vi "main(Test DQMH modules).vi"() -> ()   [LabVIEW 2018, in "Application.lvlib"] (continued)
                n5658 = To Variant(anything=T4."demux1_10_channel5" ("demux1_10(x6)_encode")) -> (Variant=w12358:variant)
                n5659 = To Variant(anything=bool[] [TRUE, FALSE, FALSE, FALSE, FALSE, FALSE]) -> (Variant=w12354:variant)
                n5660 = Bundle By Name(cluster=w12357, "command"="MEAS.AllRelaysOFF") -> (w12353:T9)
                n5661 = Bundle By Name(cluster=w12357, "command"="MEAS.mux10-1", "data"=w12364) -> (w12352:T9)
                n5662 = Bundle By Name(cluster=w12357, "command"="MEAS.mux6_1", "data"=w12362) -> (w12351:T9)
                n5663 = Bundle By Name(cluster=w12357, "command"="MEAS.demux1-10", "data"=w12358) -> (w12350:T9)
                n5664 = Bundle By Name(cluster=w12357, "command"="MEAS.eMIC", "data"=w12354) -> (w12349:T9)
                n5665 = Build Array(w12353, w12352, w12351, w12350, w12349) -> (w12334:T9[])
                n5666 = To Variant(anything=w12339) -> (Variant=w12337:variant)
                n5667 = To Variant(anything=w12339) -> (Variant=w12336:variant)
                n5668 = Bundle By Name(cluster=w12335, "command"="WaitFor") -> (w12333:T9)
                n5669 = Bundle By Name(cluster=w12335, "command"="MEAS.DMM dual read") -> (w12346:T9)
                n5670 = Bundle By Name(cluster=w12335, "command"="MEAS.requestAC", "data"=w12337) -> (w12345:T9)
                n5671 = Bundle By Name(cluster=w12335, "command"="Apps.WaitForEvent", "data"=w12336) -> (w12340:T9)
                n5672 = Bundle By Name(cluster=w12335, "command"="Apps.UI Update 1") -> (w12341:T9)
                n5673 = Build Array (concatenate)(w12334, w12333, w12346, w12345, w12340, w12341) -> (w12338:T9[])
              }
            }
          }
          frame True {
            n5674 = Bundle By Name(cluster=T9 {"command"="", "data"=variant} ("element"), "command"="Apps.UI Update 1") -> (w12368:T9)
            n5675 = Build Array(w12368) -> (w12367:T9[])
          }
        }
        n5676 = for {
          tunnel: w12283 -> [w12378] mode=indexing
          tunnel: w12291 -> [w12379]
          tunnel: [w12375] -> w12293 mode=indexing
          n5677 = Unbundle By Name(w12378) -> ("command"=w12377:string, "data"=w12376:variant)
          n5678 = call "App enquece.vi"("command data"=w12376, "command"=w12377, "queue in"=w12379) -> ("error out"=w12375:errorcluster)  [unwired: 7 in, 1 out]
        }
        n5679 = Merge Errors(w12294, w12293) -> (w12292:errorcluster)
      }
      frame "Test DRV 26A" {
        w12383 = 26 ("DUT index(0-59)")
        n5680 = disable-structure shown="LOGGING==TRUE" {
          disable-tunnel: w12388 -> [w12471 _]
          frame condition #0 (active) {
            n5681 = Empty String/Path?(string/path=w12471) -> (empty?=w12473:bool)
            n5682 = Select(t="Quece timeout", s=w12473, f=w12471) -> (s? t:f=w12470:string)
            n5683 = call "string log (SubVI).vi"("state Name"=w12470) -> ()  [unwired: 9 in, 2 out]
          }
          frame condition #1 {
          }
        }
        n5684 = Flush Queue(queue=w12389) -> (queue out=w12390:refnum<queue>)  [unwired: 1 in, 2 out]
        n5685 = Decrement(x=w12383) -> (x-1=w12387:i32)
        n5686 = Index Array(array=w12384, index=w12387) -> (element=w12385:refnum<vi>)
        n5687 = call "FGV DRV stand.vi"() -> ("Sub-Test.DCV"=w12380:bool)  [unwired: 10 in, 1 out]
        n5688 = call "FGV Driver Data.vi"("DUT index(1-60)"=w12383) -> ("DUT SC"=w12381:bool)  [unwired: 7 in, 3 out]
        n5689 = property class="ColBox"(reference=w12385, "Value"=u32 10000536 ("DRV 1")) -> ()  [unwired: 1 in, 2 out]
        n5690 = case shown="False" w12381 {
          tunnel: w12383 -> [w12401 _]
          tunnel: [w12400 w12466] -> w12382
          tunnel: w12380 -> [w12399 _]
          frame False {
            n5691 = case shown="False" w12399 {
              tunnel: w12401 -> [w12408 w12438]
              tunnel: [w12419 w12437] -> w12400
              frame False {
                w12405 = T9 {"command"="", "data"=variant} ("element")
                w12418 = T9 {"command"="", "data"=variant} ("element")
                n5692 = To Variant(anything=T3."mux10_1_channel5" ("mux10_1(x6)_encode")) -> (Variant=w12416:variant)
                n5693 = To Variant(anything=T4."demux1_10_channel5" ("demux1_10(x6)_encode")) -> (Variant=w12412:variant)
                n5694 = To Variant(anything=bool[] [FALSE, TRUE, FALSE, FALSE, FALSE, FALSE]) -> (Variant=w12427:variant)
                n5695 = Bundle By Name(cluster=w12418, "command"="MEAS.AllRelaysOFF") -> (w12426:T9)
                n5696 = Bundle By Name(cluster=w12418, "command"="MEAS.mux10-1", "data"=w12416) -> (w12409:T9)
                n5697 = Bundle By Name(cluster=w12418, "command"="MEAS.demux1-10", "data"=w12412) -> (w12410:T9)
                n5698 = Bundle By Name(cluster=w12418, "command"="MEAS.eMIC", "data"=w12427) -> (w12411:T9)
                n5699 = Build Array(w12426, w12409, w12410, w12411) -> (w12404:T9[])
                n5700 = To Variant(anything=w12408) -> (Variant=w12407:variant)
                n5701 = To Variant(anything=w12408) -> (Variant=w12406:variant)
                n5702 = Bundle By Name(cluster=w12405, "command"="MEAS.requestAC", "data"=w12407) -> (w12424:T9)
                n5703 = Bundle By Name(cluster=w12405, "command"="Apps.WaitForEvent", "data"=w12406) -> (w12420:T9)
                n5704 = Bundle By Name(cluster=w12405, "command"="Apps.UI Update 1") -> (w12421:T9)
                n5705 = Bundle By Name(cluster=w12405, "command"="WaitFor") -> (w12403:T9)
                n5706 = Build Array (concatenate)(w12404, w12403, w12424, w12420, w12421) -> (w12419:T9[])
              }
              frame True {
                w12434 = T9 {"command"="", "data"=variant} ("element")
                w12456 = T9 {"command"="", "data"=variant} ("element")
                n5707 = To Variant(anything=T3."mux10_1_channel5" ("mux10_1(x6)_encode")) -> (Variant=w12463:variant)
                n5708 = To Variant(anything=T2."mux6_1_channel2_3" ("mux6_1(3wires)_encode")) -> (Variant=w12461:variant)
                n5709 = To Variant(anything=T4."demux1_10_channel5" ("demux1_10(x6)_encode")) -> (Variant=w12457:variant)
                n5710 = To Variant(anything=bool[] [FALSE, TRUE, FALSE, FALSE, FALSE, FALSE]) -> (Variant=w12453:variant)
                n5711 = Bundle By Name(cluster=w12456, "command"="MEAS.AllRelaysOFF") -> (w12452:T9)
                n5712 = Bundle By Name(cluster=w12456, "command"="MEAS.mux10-1", "data"=w12463) -> (w12451:T9)
                n5713 = Bundle By Name(cluster=w12456, "command"="MEAS.mux6_1", "data"=w12461) -> (w12450:T9)
                n5714 = Bundle By Name(cluster=w12456, "command"="MEAS.demux1-10", "data"=w12457) -> (w12449:T9)
                n5715 = Bundle By Name(cluster=w12456, "command"="MEAS.eMIC", "data"=w12453) -> (w12448:T9)
                n5716 = Build Array(w12452, w12451, w12450, w12449, w12448) -> (w12433:T9[])
                n5717 = To Variant(anything=w12438) -> (Variant=w12436:variant)
                n5718 = To Variant(anything=w12438) -> (Variant=w12435:variant)
                n5719 = Bundle By Name(cluster=w12434, "command"="WaitFor") -> (w12432:T9)
                n5720 = Bundle By Name(cluster=w12434, "command"="MEAS.DMM dual read") -> (w12445:T9)
                n5721 = Bundle By Name(cluster=w12434, "command"="MEAS.requestAC", "data"=w12436) -> (w12444:T9)
                n5722 = Bundle By Name(cluster=w12434, "command"="Apps.WaitForEvent", "data"=w12435) -> (w12439:T9)
                n5723 = Bundle By Name(cluster=w12434, "command"="Apps.UI Update 1") -> (w12440:T9)
                n5724 = Build Array (concatenate)(w12433, w12432, w12445, w12444, w12439, w12440) -> (w12437:T9[])
              }
            }
          }
          frame True {
            n5725 = Bundle By Name(cluster=T9 {"command"="", "data"=variant} ("element"), "command"="Apps.UI Update 1") -> (w12467:T9)
            n5726 = Build Array(w12467) -> (w12466:T9[])
          }
        }
        n5727 = for {
          tunnel: w12382 -> [w12477] mode=indexing
          tunnel: w12390 -> [w12478]
          tunnel: [w12474] -> w12392 mode=indexing
          n5728 = Unbundle By Name(w12477) -> ("command"=w12476:string, "data"=w12475:variant)
          n5729 = call "App enquece.vi"("command data"=w12475, "command"=w12476, "queue in"=w12478) -> ("error out"=w12474:errorcluster)  [unwired: 7 in, 1 out]
        }
        n5730 = Merge Errors(w12393, w12392) -> (w12391:errorcluster)
      }
      frame "Test DRV 27A" {
        w12482 = 27 ("DUT index(0-59)")
        n5731 = disable-structure shown="LOGGING==TRUE" {
          disable-tunnel: w12487 -> [w12570 _]
          frame condition #0 (active) {
            n5732 = Empty String/Path?(string/path=w12570) -> (empty?=w12572:bool)
            n5733 = Select(t="Quece timeout", s=w12572, f=w12570) -> (s? t:f=w12569:string)
            n5734 = call "string log (SubVI).vi"("state Name"=w12569) -> ()  [unwired: 9 in, 2 out]
          }
          frame condition #1 {
          }
        }
        n5735 = Flush Queue(queue=w12488) -> (queue out=w12489:refnum<queue>)  [unwired: 1 in, 2 out]
        n5736 = Decrement(x=w12482) -> (x-1=w12486:i32)
        n5737 = Index Array(array=w12483, index=w12486) -> (element=w12484:refnum<vi>)
        n5738 = call "FGV DRV stand.vi"() -> ("Sub-Test.DCV"=w12479:bool)  [unwired: 10 in, 1 out]
        n5739 = call "FGV Driver Data.vi"("DUT index(1-60)"=w12482) -> ("DUT SC"=w12480:bool)  [unwired: 7 in, 3 out]
        n5740 = property class="ColBox"(reference=w12484, "Value"=u32 10000536 ("DRV 1")) -> ()  [unwired: 1 in, 2 out]
        n5741 = case shown="False" w12480 {
          tunnel: w12482 -> [w12500 _]
          tunnel: [w12499 w12565] -> w12481
          tunnel: w12479 -> [w12498 _]
          frame False {
            n5742 = case shown="True" w12498 {
              tunnel: w12500 -> [w12507 w12537]
              tunnel: [w12518 w12536] -> w12499
              frame False {
                w12504 = T9 {"command"="", "data"=variant} ("element")
                w12517 = T9 {"command"="", "data"=variant} ("element")
                n5743 = To Variant(anything=T3."mux10_1_channel5" ("mux10_1(x6)_encode")) -> (Variant=w12515:variant)
                n5744 = To Variant(anything=T4."demux1_10_channel5" ("demux1_10(x6)_encode")) -> (Variant=w12511:variant)
                n5745 = To Variant(anything=bool[] [FALSE, FALSE, TRUE, FALSE, FALSE, FALSE]) -> (Variant=w12526:variant)
                n5746 = Bundle By Name(cluster=w12517, "command"="MEAS.AllRelaysOFF") -> (w12525:T9)
                n5747 = Bundle By Name(cluster=w12517, "command"="MEAS.mux10-1", "data"=w12515) -> (w12508:T9)
                n5748 = Bundle By Name(cluster=w12517, "command"="MEAS.demux1-10", "data"=w12511) -> (w12509:T9)
                n5749 = Bundle By Name(cluster=w12517, "command"="MEAS.eMIC", "data"=w12526) -> (w12510:T9)
                n5750 = Build Array(w12525, w12508, w12509, w12510) -> (w12503:T9[])
                n5751 = To Variant(anything=w12507) -> (Variant=w12506:variant)
                n5752 = To Variant(anything=w12507) -> (Variant=w12505:variant)
                n5753 = Bundle By Name(cluster=w12504, "command"="MEAS.requestAC", "data"=w12506) -> (w12523:T9)
                n5754 = Bundle By Name(cluster=w12504, "command"="Apps.WaitForEvent", "data"=w12505) -> (w12519:T9)
                n5755 = Bundle By Name(cluster=w12504, "command"="Apps.UI Update 1") -> (w12520:T9)
                n5756 = Bundle By Name(cluster=w12504, "command"="WaitFor") -> (w12502:T9)
                n5757 = Build Array (concatenate)(w12503, w12502, w12523, w12519, w12520) -> (w12518:T9[])
              }
              frame True {
                w12533 = T9 {"command"="", "data"=variant} ("element")
                w12555 = T9 {"command"="", "data"=variant} ("element")
                n5758 = To Variant(anything=T3."mux10_1_channel5" ("mux10_1(x6)_encode")) -> (Variant=w12562:variant)
                n5759 = To Variant(anything=T2."mux6_1_channel3_3" ("mux6_1(3wires)_encode")) -> (Variant=w12560:variant)
                n5760 = To Variant(anything=T4."demux1_10_channel5" ("demux1_10(x6)_encode")) -> (Variant=w12556:variant)
                n5761 = To Variant(anything=bool[] [FALSE, FALSE, TRUE, FALSE, FALSE, FALSE]) -> (Variant=w12552:variant)
                n5762 = Bundle By Name(cluster=w12555, "command"="MEAS.AllRelaysOFF") -> (w12551:T9)
                n5763 = Bundle By Name(cluster=w12555, "command"="MEAS.mux10-1", "data"=w12562) -> (w12550:T9)
                n5764 = Bundle By Name(cluster=w12555, "command"="MEAS.mux6_1", "data"=w12560) -> (w12549:T9)
                n5765 = Bundle By Name(cluster=w12555, "command"="MEAS.demux1-10", "data"=w12556) -> (w12548:T9)
                n5766 = Bundle By Name(cluster=w12555, "command"="MEAS.eMIC", "data"=w12552) -> (w12547:T9)
                n5767 = Build Array(w12551, w12550, w12549, w12548, w12547) -> (w12532:T9[])
                n5768 = To Variant(anything=w12537) -> (Variant=w12535:variant)
                n5769 = To Variant(anything=w12537) -> (Variant=w12534:variant)
                n5770 = Bundle By Name(cluster=w12533, "command"="WaitFor") -> (w12531:T9)
                n5771 = Bundle By Name(cluster=w12533, "command"="MEAS.DMM dual read") -> (w12544:T9)
                n5772 = Bundle By Name(cluster=w12533, "command"="MEAS.requestAC", "data"=w12535) -> (w12543:T9)
                n5773 = Bundle By Name(cluster=w12533, "command"="Apps.WaitForEvent", "data"=w12534) -> (w12538:T9)
                n5774 = Bundle By Name(cluster=w12533, "command"="Apps.UI Update 1") -> (w12539:T9)
                n5775 = Build Array (concatenate)(w12532, w12531, w12544, w12543, w12538, w12539) -> (w12536:T9[])
              }
            }
          }
          frame True {
            n5776 = Bundle By Name(cluster=T9 {"command"="", "data"=variant} ("element"), "command"="Apps.UI Update 1") -> (w12566:T9)
            n5777 = Build Array(w12566) -> (w12565:T9[])
          }
        }
        n5778 = for {
          tunnel: w12481 -> [w12576] mode=indexing
          tunnel: w12489 -> [w12577]
          tunnel: [w12573] -> w12491 mode=indexing
          n5779 = Unbundle By Name(w12576) -> ("command"=w12575:string, "data"=w12574:variant)
          n5780 = call "App enquece.vi"("command data"=w12574, "command"=w12575, "queue in"=w12577) -> ("error out"=w12573:errorcluster)  [unwired: 7 in, 1 out]
        }
        n5781 = Merge Errors(w12492, w12491) -> (w12490:errorcluster)
      }
      frame "Test DRV 28A" {
        w12581 = 28 ("DUT index(0-59)")
        n5782 = disable-structure shown="LOGGING==TRUE" {
          disable-tunnel: w12586 -> [w12669 _]
          frame condition #0 (active) {
            n5783 = Empty String/Path?(string/path=w12669) -> (empty?=w12671:bool)
            n5784 = Select(t="Quece timeout", s=w12671, f=w12669) -> (s? t:f=w12668:string)
            n5785 = call "string log (SubVI).vi"("state Name"=w12668) -> ()  [unwired: 9 in, 2 out]
          }
          frame condition #1 {
          }
        }
        n5786 = Flush Queue(queue=w12587) -> (queue out=w12588:refnum<queue>)  [unwired: 1 in, 2 out]
        n5787 = Decrement(x=w12581) -> (x-1=w12585:i32)
        n5788 = Index Array(array=w12582, index=w12585) -> (element=w12583:refnum<vi>)
        n5789 = call "FGV DRV stand.vi"() -> ("Sub-Test.DCV"=w12578:bool)  [unwired: 10 in, 1 out]
        n5790 = call "FGV Driver Data.vi"("DUT index(1-60)"=w12581) -> ("DUT SC"=w12579:bool)  [unwired: 7 in, 3 out]
        n5791 = property class="ColBox"(reference=w12583, "Value"=u32 10000536 ("DRV 1")) -> ()  [unwired: 1 in, 2 out]
        n5792 = case shown="False" w12579 {
          tunnel: w12581 -> [w12599 _]
          tunnel: [w12598 w12664] -> w12580
          tunnel: w12578 -> [w12597 _]
          frame False {
            n5793 = case shown="False" w12597 {
              tunnel: w12599 -> [w12606 w12636]
              tunnel: [w12617 w12635] -> w12598
              frame False {
                w12603 = T9 {"command"="", "data"=variant} ("element")
                w12616 = T9 {"command"="", "data"=variant} ("element")
                n5794 = To Variant(anything=T3."mux10_1_channel5" ("mux10_1(x6)_encode")) -> (Variant=w12614:variant)
                n5795 = To Variant(anything=T4."demux1_10_channel5" ("demux1_10(x6)_encode")) -> (Variant=w12610:variant)
                n5796 = To Variant(anything=bool[] [FALSE, FALSE, FALSE, TRUE, FALSE, FALSE]) -> (Variant=w12625:variant)
                n5797 = Bundle By Name(cluster=w12616, "command"="MEAS.AllRelaysOFF") -> (w12624:T9)
                n5798 = Bundle By Name(cluster=w12616, "command"="MEAS.mux10-1", "data"=w12614) -> (w12607:T9)
                n5799 = Bundle By Name(cluster=w12616, "command"="MEAS.demux1-10", "data"=w12610) -> (w12608:T9)
                n5800 = Bundle By Name(cluster=w12616, "command"="MEAS.eMIC", "data"=w12625) -> (w12609:T9)
                n5801 = Build Array(w12624, w12607, w12608, w12609) -> (w12602:T9[])
                n5802 = To Variant(anything=w12606) -> (Variant=w12605:variant)
                n5803 = To Variant(anything=w12606) -> (Variant=w12604:variant)
                n5804 = Bundle By Name(cluster=w12603, "command"="MEAS.requestAC", "data"=w12605) -> (w12622:T9)
                n5805 = Bundle By Name(cluster=w12603, "command"="Apps.WaitForEvent", "data"=w12604) -> (w12618:T9)
                n5806 = Bundle By Name(cluster=w12603, "command"="Apps.UI Update 1") -> (w12619:T9)
                n5807 = Bundle By Name(cluster=w12603, "command"="WaitFor") -> (w12601:T9)
                n5808 = Build Array (concatenate)(w12602, w12601, w12622, w12618, w12619) -> (w12617:T9[])
              }
              frame True {
                w12632 = T9 {"command"="", "data"=variant} ("element")
                w12654 = T9 {"command"="", "data"=variant} ("element")
                n5809 = To Variant(anything=T3."mux10_1_channel5" ("mux10_1(x6)_encode")) -> (Variant=w12661:variant)
                n5810 = To Variant(anything=T2."mux6_1_channel4_3" ("mux6_1(3wires)_encode")) -> (Variant=w12659:variant)
                n5811 = To Variant(anything=T4."demux1_10_channel5" ("demux1_10(x6)_encode")) -> (Variant=w12655:variant)
                n5812 = To Variant(anything=bool[] [FALSE, FALSE, FALSE, TRUE, FALSE, FALSE]) -> (Variant=w12651:variant)
                n5813 = Bundle By Name(cluster=w12654, "command"="MEAS.AllRelaysOFF") -> (w12650:T9)
                n5814 = Bundle By Name(cluster=w12654, "command"="MEAS.mux10-1", "data"=w12661) -> (w12649:T9)
                n5815 = Bundle By Name(cluster=w12654, "command"="MEAS.mux6_1", "data"=w12659) -> (w12648:T9)
                n5816 = Bundle By Name(cluster=w12654, "command"="MEAS.demux1-10", "data"=w12655) -> (w12647:T9)
                n5817 = Bundle By Name(cluster=w12654, "command"="MEAS.eMIC", "data"=w12651) -> (w12646:T9)
                n5818 = Build Array(w12650, w12649, w12648, w12647, w12646) -> (w12631:T9[])
                n5819 = To Variant(anything=w12636) -> (Variant=w12634:variant)
                n5820 = To Variant(anything=w12636) -> (Variant=w12633:variant)
                n5821 = Bundle By Name(cluster=w12632, "command"="WaitFor") -> (w12630:T9)
                n5822 = Bundle By Name(cluster=w12632, "command"="MEAS.DMM dual read") -> (w12643:T9)
                n5823 = Bundle By Name(cluster=w12632, "command"="MEAS.requestAC", "data"=w12634) -> (w12642:T9)
                n5824 = Bundle By Name(cluster=w12632, "command"="Apps.WaitForEvent", "data"=w12633) -> (w12637:T9)
                n5825 = Bundle By Name(cluster=w12632, "command"="Apps.UI Update 1") -> (w12638:T9)
                n5826 = Build Array (concatenate)(w12631, w12630, w12643, w12642, w12637, w12638) -> (w12635:T9[])
              }
            }
          }
          frame True {
            n5827 = Bundle By Name(cluster=T9 {"command"="", "data"=variant} ("element"), "command"="Apps.UI Update 1") -> (w12665:T9)
            n5828 = Build Array(w12665) -> (w12664:T9[])
          }
        }
        n5829 = for {
          tunnel: w12580 -> [w12675] mode=indexing
          tunnel: w12588 -> [w12676]
          tunnel: [w12672] -> w12590 mode=indexing
          n5830 = Unbundle By Name(w12675) -> ("command"=w12674:string, "data"=w12673:variant)
          n5831 = call "App enquece.vi"("command data"=w12673, "command"=w12674, "queue in"=w12676) -> ("error out"=w12672:errorcluster)  [unwired: 7 in, 1 out]
        }
        n5832 = Merge Errors(w12591, w12590) -> (w12589:errorcluster)
      }
      frame "Test DRV 29A" {
        w12680 = 29 ("DUT index(0-59)")
        n5833 = disable-structure shown="LOGGING==TRUE" {
          disable-tunnel: w12685 -> [w12768 _]
          frame condition #0 (active) {
            n5834 = Empty String/Path?(string/path=w12768) -> (empty?=w12770:bool)
            n5835 = Select(t="Quece timeout", s=w12770, f=w12768) -> (s? t:f=w12767:string)
            n5836 = call "string log (SubVI).vi"("state Name"=w12767) -> ()  [unwired: 9 in, 2 out]
          }
          frame condition #1 {
          }
        }
        n5837 = Flush Queue(queue=w12686) -> (queue out=w12687:refnum<queue>)  [unwired: 1 in, 2 out]
        n5838 = Decrement(x=w12680) -> (x-1=w12684:i32)
        n5839 = Index Array(array=w12681, index=w12684) -> (element=w12682:refnum<vi>)
        n5840 = call "FGV DRV stand.vi"() -> ("Sub-Test.DCV"=w12677:bool)  [unwired: 10 in, 1 out]
        n5841 = call "FGV Driver Data.vi"("DUT index(1-60)"=w12680) -> ("DUT SC"=w12678:bool)  [unwired: 7 in, 3 out]
        n5842 = property class="ColBox"(reference=w12682, "Value"=u32 10000536 ("DRV 1")) -> ()  [unwired: 1 in, 2 out]
        n5843 = case shown="False" w12678 {
          tunnel: w12680 -> [w12698 _]
          tunnel: [w12697 w12763] -> w12679
          tunnel: w12677 -> [w12696 _]
          frame False {
            n5844 = case shown="True" w12696 {
              tunnel: w12698 -> [w12705 w12735]
              tunnel: [w12716 w12734] -> w12697
              frame False {
                w12702 = T9 {"command"="", "data"=variant} ("element")
                w12715 = T9 {"command"="", "data"=variant} ("element")
                n5845 = To Variant(anything=T3."mux10_1_channel5" ("mux10_1(x6)_encode")) -> (Variant=w12713:variant)
                n5846 = To Variant(anything=T4."demux1_10_channel5" ("demux1_10(x6)_encode")) -> (Variant=w12709:variant)
                n5847 = To Variant(anything=bool[] [FALSE, FALSE, FALSE, FALSE, TRUE, FALSE]) -> (Variant=w12724:variant)
                n5848 = Bundle By Name(cluster=w12715, "command"="MEAS.AllRelaysOFF") -> (w12723:T9)
                n5849 = Bundle By Name(cluster=w12715, "command"="MEAS.mux10-1", "data"=w12713) -> (w12706:T9)
                n5850 = Bundle By Name(cluster=w12715, "command"="MEAS.demux1-10", "data"=w12709) -> (w12707:T9)
                n5851 = Bundle By Name(cluster=w12715, "command"="MEAS.eMIC", "data"=w12724) -> (w12708:T9)
                n5852 = Build Array(w12723, w12706, w12707, w12708) -> (w12701:T9[])
                n5853 = To Variant(anything=w12705) -> (Variant=w12704:variant)
                n5854 = To Variant(anything=w12705) -> (Variant=w12703:variant)
                n5855 = Bundle By Name(cluster=w12702, "command"="MEAS.requestAC", "data"=w12704) -> (w12721:T9)
                n5856 = Bundle By Name(cluster=w12702, "command"="Apps.WaitForEvent", "data"=w12703) -> (w12717:T9)
                n5857 = Bundle By Name(cluster=w12702, "command"="Apps.UI Update 1") -> (w12718:T9)
                n5858 = Bundle By Name(cluster=w12702, "command"="WaitFor") -> (w12700:T9)
                n5859 = Build Array (concatenate)(w12701, w12700, w12721, w12717, w12718) -> (w12716:T9[])
              }
              frame True {
                w12731 = T9 {"command"="", "data"=variant} ("element")
                w12753 = T9 {"command"="", "data"=variant} ("element")
                n5860 = To Variant(anything=T3."mux10_1_channel5" ("mux10_1(x6)_encode")) -> (Variant=w12760:variant)
                n5861 = To Variant(anything=T2."mux6_1_channel5_3" ("mux6_1(3wires)_encode")) -> (Variant=w12758:variant)
                n5862 = To Variant(anything=T4."demux1_10_channel5" ("demux1_10(x6)_encode")) -> (Variant=w12754:variant)
                n5863 = To Variant(anything=bool[] [FALSE, FALSE, FALSE, FALSE, TRUE, FALSE]) -> (Variant=w12750:variant)
                n5864 = Bundle By Name(cluster=w12753, "command"="MEAS.AllRelaysOFF") -> (w12749:T9)
                n5865 = Bundle By Name(cluster=w12753, "command"="MEAS.mux10-1", "data"=w12760) -> (w12748:T9)
                n5866 = Bundle By Name(cluster=w12753, "command"="MEAS.mux6_1", "data"=w12758) -> (w12747:T9)
                n5867 = Bundle By Name(cluster=w12753, "command"="MEAS.demux1-10", "data"=w12754) -> (w12746:T9)
                n5868 = Bundle By Name(cluster=w12753, "command"="MEAS.eMIC", "data"=w12750) -> (w12745:T9)
                n5869 = Build Array(w12749, w12748, w12747, w12746, w12745) -> (w12730:T9[])
                n5870 = To Variant(anything=w12735) -> (Variant=w12733:variant)
                n5871 = To Variant(anything=w12735) -> (Variant=w12732:variant)
                n5872 = Bundle By Name(cluster=w12731, "command"="WaitFor") -> (w12729:T9)
                n5873 = Bundle By Name(cluster=w12731, "command"="MEAS.DMM dual read") -> (w12742:T9)
                n5874 = Bundle By Name(cluster=w12731, "command"="MEAS.requestAC", "data"=w12733) -> (w12741:T9)
                n5875 = Bundle By Name(cluster=w12731, "command"="Apps.WaitForEvent", "data"=w12732) -> (w12736:T9)
                n5876 = Bundle By Name(cluster=w12731, "command"="Apps.UI Update 1") -> (w12737:T9)
                n5877 = Build Array (concatenate)(w12730, w12729, w12742, w12741, w12736, w12737) -> (w12734:T9[])
              }
            }
          }
          frame True {
            n5878 = Bundle By Name(cluster=T9 {"command"="", "data"=variant} ("element"), "command"="Apps.UI Update 1") -> (w12764:T9)
            n5879 = Build Array(w12764) -> (w12763:T9[])
          }
        }
        n5880 = for {
          tunnel: w12679 -> [w12774] mode=indexing
          tunnel: w12687 -> [w12775]
          tunnel: [w12771] -> w12689 mode=indexing
          n5881 = Unbundle By Name(w12774) -> ("command"=w12773:string, "data"=w12772:variant)
          n5882 = call "App enquece.vi"("command data"=w12772, "command"=w12773, "queue in"=w12775) -> ("error out"=w12771:errorcluster)  [unwired: 7 in, 1 out]
        }
        n5883 = Merge Errors(w12690, w12689) -> (w12688:errorcluster)
      }
      frame "Test DRV 30A" {
        w12779 = 30 ("DUT index(0-59)")
        n5884 = disable-structure shown="LOGGING==TRUE" {
          disable-tunnel: w12784 -> [w12867 _]
          frame condition #0 (active) {
            n5885 = Empty String/Path?(string/path=w12867) -> (empty?=w12869:bool)
            n5886 = Select(t="Quece timeout", s=w12869, f=w12867) -> (s? t:f=w12866:string)
            n5887 = call "string log (SubVI).vi"("state Name"=w12866) -> ()  [unwired: 9 in, 2 out]
          }
          frame condition #1 {
          }
        }
        n5888 = Flush Queue(queue=w12785) -> (queue out=w12786:refnum<queue>)  [unwired: 1 in, 2 out]
        n5889 = Decrement(x=w12779) -> (x-1=w12783:i32)
        n5890 = Index Array(array=w12780, index=w12783) -> (element=w12781:refnum<vi>)
        n5891 = call "FGV DRV stand.vi"() -> ("Sub-Test.DCV"=w12776:bool)  [unwired: 10 in, 1 out]
        n5892 = call "FGV Driver Data.vi"("DUT index(1-60)"=w12779) -> ("DUT SC"=w12777:bool)  [unwired: 7 in, 3 out]
        n5893 = property class="ColBox"(reference=w12781, "Value"=u32 10000536 ("DRV 1")) -> ()  [unwired: 1 in, 2 out]
        n5894 = case shown="False" w12777 {
          tunnel: w12779 -> [w12797 _]
          tunnel: [w12796 w12862] -> w12778
          tunnel: w12776 -> [w12795 _]
          frame False {
            n5895 = case shown="False" w12795 {
              tunnel: w12797 -> [w12804 w12834]
              tunnel: [w12815 w12833] -> w12796
              frame False {
                w12801 = T9 {"command"="", "data"=variant} ("element")
                w12814 = T9 {"command"="", "data"=variant} ("element")
                n5896 = To Variant(anything=T3."mux10_1_channel5" ("mux10_1(x6)_encode")) -> (Variant=w12812:variant)
                n5897 = To Variant(anything=T4."demux1_10_channel5" ("demux1_10(x6)_encode")) -> (Variant=w12808:variant)
                n5898 = To Variant(anything=bool[] [FALSE, FALSE, FALSE, FALSE, FALSE, TRUE]) -> (Variant=w12823:variant)
                n5899 = Bundle By Name(cluster=w12814, "command"="MEAS.AllRelaysOFF") -> (w12822:T9)
                n5900 = Bundle By Name(cluster=w12814, "command"="MEAS.mux10-1", "data"=w12812) -> (w12805:T9)
                n5901 = Bundle By Name(cluster=w12814, "command"="MEAS.demux1-10", "data"=w12808) -> (w12806:T9)
                n5902 = Bundle By Name(cluster=w12814, "command"="MEAS.eMIC", "data"=w12823) -> (w12807:T9)
                n5903 = Build Array(w12822, w12805, w12806, w12807) -> (w12800:T9[])
                n5904 = To Variant(anything=w12804) -> (Variant=w12803:variant)
                n5905 = To Variant(anything=w12804) -> (Variant=w12802:variant)
                n5906 = Bundle By Name(cluster=w12801, "command"="MEAS.requestAC", "data"=w12803) -> (w12820:T9)
                n5907 = Bundle By Name(cluster=w12801, "command"="Apps.WaitForEvent", "data"=w12802) -> (w12816:T9)
                n5908 = Bundle By Name(cluster=w12801, "command"="Apps.UI Update 1") -> (w12817:T9)
                n5909 = Bundle By Name(cluster=w12801, "command"="WaitFor") -> (w12799:T9)
                n5910 = Build Array (concatenate)(w12800, w12799, w12820, w12816, w12817) -> (w12815:T9[])
              }
              frame True {
                w12830 = T9 {"command"="", "data"=variant} ("element")
                w12852 = T9 {"command"="", "data"=variant} ("element")
                n5911 = To Variant(anything=T3."mux10_1_channel5" ("mux10_1(x6)_encode")) -> (Variant=w12859:variant)
                n5912 = To Variant(anything=T2."mux6_1_channel6_3" ("mux6_1(3wires)_encode")) -> (Variant=w12857:variant)
                n5913 = To Variant(anything=T4."demux1_10_channel5" ("demux1_10(x6)_encode")) -> (Variant=w12853:variant)
                n5914 = To Variant(anything=bool[] [FALSE, FALSE, FALSE, FALSE, FALSE, TRUE]) -> (Variant=w12849:variant)
                n5915 = Bundle By Name(cluster=w12852, "command"="MEAS.AllRelaysOFF") -> (w12848:T9)
                n5916 = Bundle By Name(cluster=w12852, "command"="MEAS.mux10-1", "data"=w12859) -> (w12847:T9)
                n5917 = Bundle By Name(cluster=w12852, "command"="MEAS.mux6_1", "data"=w12857) -> (w12846:T9)
                n5918 = Bundle By Name(cluster=w12852, "command"="MEAS.demux1-10", "data"=w12853) -> (w12845:T9)
                n5919 = Bundle By Name(cluster=w12852, "command"="MEAS.eMIC", "data"=w12849) -> (w12844:T9)
                n5920 = Build Array(w12848, w12847, w12846, w12845, w12844) -> (w12829:T9[])
                n5921 = To Variant(anything=w12834) -> (Variant=w12832:variant)
                n5922 = To Variant(anything=w12834) -> (Variant=w12831:variant)
                n5923 = Bundle By Name(cluster=w12830, "command"="WaitFor") -> (w12828:T9)
                n5924 = Bundle By Name(cluster=w12830, "command"="MEAS.DMM dual read") -> (w12841:T9)
                n5925 = Bundle By Name(cluster=w12830, "command"="MEAS.requestAC", "data"=w12832) -> (w12840:T9)
                n5926 = Bundle By Name(cluster=w12830, "command"="Apps.WaitForEvent", "data"=w12831) -> (w12835:T9)
                n5927 = Bundle By Name(cluster=w12830, "command"="Apps.UI Update 1") -> (w12836:T9)
                n5928 = Build Array (concatenate)(w12829, w12828, w12841, w12840, w12835, w12836) -> (w12833:T9[])
              }
            }
          }
          frame True {
            n5929 = Bundle By Name(cluster=T9 {"command"="", "data"=variant} ("element"), "command"="Apps.UI Update 1") -> (w12863:T9)
            n5930 = Build Array(w12863) -> (w12862:T9[])
          }
        }
        n5931 = for {
          tunnel: w12778 -> [w12873] mode=indexing
          tunnel: w12786 -> [w12874]
          tunnel: [w12870] -> w12788 mode=indexing
          n5932 = Unbundle By Name(w12873) -> ("command"=w12872:string, "data"=w12871:variant)
          n5933 = call "App enquece.vi"("command data"=w12871, "command"=w12872, "queue in"=w12874) -> ("error out"=w12870:errorcluster)  [unwired: 7 in, 1 out]
        }
        n5934 = Merge Errors(w12789, w12788) -> (w12787:errorcluster)
      }
      frame "Test DRV 31A" {
        w12878 = 31 ("DUT index(0-59)")
        n5935 = disable-structure shown="LOGGING==TRUE" {
          disable-tunnel: w12883 -> [w12966 _]
          frame condition #0 (active) {
            n5936 = Empty String/Path?(string/path=w12966) -> (empty?=w12968:bool)
            n5937 = Select(t="Quece timeout", s=w12968, f=w12966) -> (s? t:f=w12965:string)
            n5938 = call "string log (SubVI).vi"("state Name"=w12965) -> ()  [unwired: 9 in, 2 out]
          }
          frame condition #1 {
          }
        }
        n5939 = Flush Queue(queue=w12884) -> (queue out=w12885:refnum<queue>)  [unwired: 1 in, 2 out]
        n5940 = Decrement(x=w12878) -> (x-1=w12882:i32)
        n5941 = Index Array(array=w12879, index=w12882) -> (element=w12880:refnum<vi>)
        n5942 = call "FGV DRV stand.vi"() -> ("Sub-Test.DCV"=w12875:bool)  [unwired: 10 in, 1 out]
        n5943 = call "FGV Driver Data.vi"("DUT index(1-60)"=w12878) -> ("DUT SC"=w12876:bool)  [unwired: 7 in, 3 out]
        n5944 = property class="ColBox"(reference=w12880, "Value"=u32 10000536 ("DRV 1")) -> ()  [unwired: 1 in, 2 out]
        n5945 = case shown="False" w12876 {
          tunnel: w12878 -> [w12896 _]
          tunnel: [w12895 w12961] -> w12877
          tunnel: w12875 -> [w12894 _]
          frame False {
            n5946 = case shown="True" w12894 {
              tunnel: w12896 -> [w12903 w12933]
              tunnel: [w12914 w12932] -> w12895
              frame False {
                w12900 = T9 {"command"="", "data"=variant} ("element")
                w12913 = T9 {"command"="", "data"=variant} ("element")
                n5947 = To Variant(anything=T3."mux10_1_channel6" ("mux10_1(x6)_encode")) -> (Variant=w12911:variant)
                n5948 = To Variant(anything=T4."demux1_10_channel6" ("demux1_10(x6)_encode")) -> (Variant=w12907:variant)
                n5949 = To Variant(anything=bool[] [TRUE, FALSE, FALSE, FALSE, FALSE, FALSE]) -> (Variant=w12922:variant)
                n5950 = Bundle By Name(cluster=w12913, "command"="MEAS.AllRelaysOFF") -> (w12921:T9)
                n5951 = Bundle By Name(cluster=w12913, "command"="MEAS.mux10-1", "data"=w12911) -> (w12904:T9)
                n5952 = Bundle By Name(cluster=w12913, "command"="MEAS.demux1-10", "data"=w12907) -> (w12905:T9)
                n5953 = Bundle By Name(cluster=w12913, "command"="MEAS.eMIC", "data"=w12922) -> (w12906:T9)
                n5954 = Build Array(w12921, w12904, w12905, w12906) -> (w12899:T9[])
                n5955 = To Variant(anything=w12903) -> (Variant=w12902:variant)
                n5956 = To Variant(anything=w12903) -> (Variant=w12901:variant)
                n5957 = Bundle By Name(cluster=w12900, "command"="MEAS.requestAC", "data"=w12902) -> (w12919:T9)
                n5958 = Bundle By Name(cluster=w12900, "command"="Apps.WaitForEvent", "data"=w12901) -> (w12915:T9)
                n5959 = Bundle By Name(cluster=w12900, "command"="Apps.UI Update 1") -> (w12916:T9)
                n5960 = Bundle By Name(cluster=w12900, "command"="WaitFor") -> (w12898:T9)
                n5961 = Build Array (concatenate)(w12899, w12898, w12919, w12915, w12916) -> (w12914:T9[])
              }
              frame True {
                w12929 = T9 {"command"="", "data"=variant} ("element")
                w12951 = T9 {"command"="", "data"=variant} ("element")
                n5962 = To Variant(anything=T3."mux10_1_channel6" ("mux10_1(x6)_encode")) -> (Variant=w12958:variant)
                n5963 = To Variant(anything=T2."mux6_1_channel1_3" ("mux6_1(3wires)_encode")) -> (Variant=w12956:variant)
                n5964 = To Variant(anything=T4."demux1_10_channel6" ("demux1_10(x6)_encode")) -> (Variant=w12952:variant)
                n5965 = To Variant(anything=bool[] [TRUE, FALSE, FALSE, FALSE, FALSE, FALSE]) -> (Variant=w12948:variant)
                n5966 = Bundle By Name(cluster=w12951, "command"="MEAS.AllRelaysOFF") -> (w12947:T9)
                n5967 = Bundle By Name(cluster=w12951, "command"="MEAS.mux10-1", "data"=w12958) -> (w12946:T9)
                n5968 = Bundle By Name(cluster=w12951, "command"="MEAS.mux6_1", "data"=w12956) -> (w12945:T9)
                n5969 = Bundle By Name(cluster=w12951, "command"="MEAS.demux1-10", "data"=w12952) -> (w12944:T9)
                n5970 = Bundle By Name(cluster=w12951, "command"="MEAS.eMIC", "data"=w12948) -> (w12943:T9)
                n5971 = Build Array(w12947, w12946, w12945, w12944, w12943) -> (w12928:T9[])
                n5972 = To Variant(anything=w12933) -> (Variant=w12931:variant)
                n5973 = To Variant(anything=w12933) -> (Variant=w12930:variant)
                n5974 = Bundle By Name(cluster=w12929, "command"="WaitFor") -> (w12927:T9)
                n5975 = Bundle By Name(cluster=w12929, "command"="MEAS.DMM dual read") -> (w12940:T9)
                n5976 = Bundle By Name(cluster=w12929, "command"="MEAS.requestAC", "data"=w12931) -> (w12939:T9)
                n5977 = Bundle By Name(cluster=w12929, "command"="Apps.WaitForEvent", "data"=w12930) -> (w12934:T9)
                n5978 = Bundle By Name(cluster=w12929, "command"="Apps.UI Update 1") -> (w12935:T9)
                n5979 = Build Array (concatenate)(w12928, w12927, w12940, w12939, w12934, w12935) -> (w12932:T9[])
              }
            }
          }
          frame True {
            n5980 = Bundle By Name(cluster=T9 {"command"="", "data"=variant} ("element"), "command"="Apps.UI Update 1") -> (w12962:T9)
            n5981 = Build Array(w12962) -> (w12961:T9[])
          }
        }
        n5982 = for {
          tunnel: w12877 -> [w12972] mode=indexing
          tunnel: w12885 -> [w12973]
          tunnel: [w12969] -> w12887 mode=indexing
          n5983 = Unbundle By Name(w12972) -> ("command"=w12971:string, "data"=w12970:variant)
          n5984 = call "App enquece.vi"("command data"=w12970, "command"=w12971, "queue in"=w12973) -> ("error out"=w12969:errorcluster)  [unwired: 7 in, 1 out]
        }
        n5985 = Merge Errors(w12888, w12887) -> (w12886:errorcluster)
      }
      frame "Test DRV 32A" {
        w12977 = 32 ("DUT index(0-59)")
        n5986 = disable-structure shown="LOGGING==TRUE" {
          disable-tunnel: w12982 -> [w13065 _]
          frame condition #0 (active) {
            n5987 = Empty String/Path?(string/path=w13065) -> (empty?=w13067:bool)
            n5988 = Select(t="Quece timeout", s=w13067, f=w13065) -> (s? t:f=w13064:string)
            n5989 = call "string log (SubVI).vi"("state Name"=w13064) -> ()  [unwired: 9 in, 2 out]
          }
          frame condition #1 {
          }
        }
        n5990 = Flush Queue(queue=w12983) -> (queue out=w12984:refnum<queue>)  [unwired: 1 in, 2 out]
        n5991 = Decrement(x=w12977) -> (x-1=w12981:i32)
        n5992 = Index Array(array=w12978, index=w12981) -> (element=w12979:refnum<vi>)
        n5993 = call "FGV DRV stand.vi"() -> ("Sub-Test.DCV"=w12974:bool)  [unwired: 10 in, 1 out]
        n5994 = call "FGV Driver Data.vi"("DUT index(1-60)"=w12977) -> ("DUT SC"=w12975:bool)  [unwired: 7 in, 3 out]
        n5995 = property class="ColBox"(reference=w12979, "Value"=u32 10000536 ("DRV 1")) -> ()  [unwired: 1 in, 2 out]
        n5996 = case shown="False" w12975 {
          tunnel: w12977 -> [w12995 _]
          tunnel: [w12994 w13060] -> w12976
          tunnel: w12974 -> [w12993 _]
          frame False {
            n5997 = case shown="False" w12993 {
              tunnel: w12995 -> [w13002 w13032]
              tunnel: [w13013 w13031] -> w12994
              frame False {
                w12999 = T9 {"command"="", "data"=variant} ("element")
                w13012 = T9 {"command"="", "data"=variant} ("element")
                n5998 = To Variant(anything=T3."mux10_1_channel6" ("mux10_1(x6)_encode")) -> (Variant=w13010:variant)
                n5999 = To Variant(anything=T4."demux1_10_channel6" ("demux1_10(x6)_encode")) -> (Variant=w13006:variant)
                n6000 = To Variant(anything=bool[] [FALSE, TRUE, FALSE, FALSE, FALSE, FALSE]) -> (Variant=w13021:variant)
                n6001 = Bundle By Name(cluster=w13012, "command"="MEAS.AllRelaysOFF") -> (w13020:T9)
                n6002 = Bundle By Name(cluster=w13012, "command"="MEAS.mux10-1", "data"=w13010) -> (w13003:T9)
                n6003 = Bundle By Name(cluster=w13012, "command"="MEAS.demux1-10", "data"=w13006) -> (w13004:T9)
                n6004 = Bundle By Name(cluster=w13012, "command"="MEAS.eMIC", "data"=w13021) -> (w13005:T9)
                n6005 = Build Array(w13020, w13003, w13004, w13005) -> (w12998:T9[])
                n6006 = To Variant(anything=w13002) -> (Variant=w13001:variant)
                n6007 = To Variant(anything=w13002) -> (Variant=w13000:variant)
                n6008 = Bundle By Name(cluster=w12999, "command"="MEAS.requestAC", "data"=w13001) -> (w13018:T9)
                n6009 = Bundle By Name(cluster=w12999, "command"="Apps.WaitForEvent", "data"=w13000) -> (w13014:T9)
                n6010 = Bundle By Name(cluster=w12999, "command"="Apps.UI Update 1") -> (w13015:T9)
                n6011 = Bundle By Name(cluster=w12999, "command"="WaitFor") -> (w12997:T9)
                n6012 = Build Array (concatenate)(w12998, w12997, w13018, w13014, w13015) -> (w13013:T9[])
              }
              frame True {
                w13028 = T9 {"command"="", "data"=variant} ("element")
                w13050 = T9 {"command"="", "data"=variant} ("element")
                n6013 = To Variant(anything=T3."mux10_1_channel6" ("mux10_1(x6)_encode")) -> (Variant=w13057:variant)
                n6014 = To Variant(anything=T2."mux6_1_channel2_3" ("mux6_1(3wires)_encode")) -> (Variant=w13055:variant)
                n6015 = To Variant(anything=T4."demux1_10_channel6" ("demux1_10(x6)_encode")) -> (Variant=w13051:variant)
                n6016 = To Variant(anything=bool[] [FALSE, TRUE, FALSE, FALSE, FALSE, FALSE]) -> (Variant=w13047:variant)
                n6017 = Bundle By Name(cluster=w13050, "command"="MEAS.AllRelaysOFF") -> (w13046:T9)
                n6018 = Bundle By Name(cluster=w13050, "command"="MEAS.mux10-1", "data"=w13057) -> (w13045:T9)
                n6019 = Bundle By Name(cluster=w13050, "command"="MEAS.mux6_1", "data"=w13055) -> (w13044:T9)
                n6020 = Bundle By Name(cluster=w13050, "command"="MEAS.demux1-10", "data"=w13051) -> (w13043:T9)
                n6021 = Bundle By Name(cluster=w13050, "command"="MEAS.eMIC", "data"=w13047) -> (w13042:T9)
                n6022 = Build Array(w13046, w13045, w13044, w13043, w13042) -> (w13027:T9[])
                n6023 = To Variant(anything=w13032) -> (Variant=w13030:variant)
                n6024 = To Variant(anything=w13032) -> (Variant=w13029:variant)
                n6025 = Bundle By Name(cluster=w13028, "command"="WaitFor") -> (w13026:T9)
                n6026 = Bundle By Name(cluster=w13028, "command"="MEAS.DMM dual read") -> (w13039:T9)
                n6027 = Bundle By Name(cluster=w13028, "command"="MEAS.requestAC", "data"=w13030) -> (w13038:T9)
                n6028 = Bundle By Name(cluster=w13028, "command"="Apps.WaitForEvent", "data"=w13029) -> (w13033:T9)
                n6029 = Bundle By Name(cluster=w13028, "command"="Apps.UI Update 1") -> (w13034:T9)
                n6030 = Build Array (concatenate)(w13027, w13026, w13039, w13038, w13033, w13034) -> (w13031:T9[])
              }
            }
          }
          frame True {
            n6031 = Bundle By Name(cluster=T9 {"command"="", "data"=variant} ("element"), "command"="Apps.UI Update 1") -> (w13061:T9)
            n6032 = Build Array(w13061) -> (w13060:T9[])
          }
        }
        n6033 = for {
          tunnel: w12976 -> [w13071] mode=indexing
          tunnel: w12984 -> [w13072]
          tunnel: [w13068] -> w12986 mode=indexing
          n6034 = Unbundle By Name(w13071) -> ("command"=w13070:string, "data"=w13069:variant)
          n6035 = call "App enquece.vi"("command data"=w13069, "command"=w13070, "queue in"=w13072) -> ("error out"=w13068:errorcluster)  [unwired: 7 in, 1 out]
        }
        n6036 = Merge Errors(w12987, w12986) -> (w12985:errorcluster)
      }
      frame "Test DRV 33A" {
        w13076 = 33 ("DUT index(0-59)")
        n6037 = disable-structure shown="LOGGING==TRUE" {
          disable-tunnel: w13081 -> [w13164 _]
          frame condition #0 (active) {
            n6038 = Empty String/Path?(string/path=w13164) -> (empty?=w13166:bool)
            n6039 = Select(t="Quece timeout", s=w13166, f=w13164) -> (s? t:f=w13163:string)
            n6040 = call "string log (SubVI).vi"("state Name"=w13163) -> ()  [unwired: 9 in, 2 out]
          }
          frame condition #1 {
          }
        }
        n6041 = Flush Queue(queue=w13082) -> (queue out=w13083:refnum<queue>)  [unwired: 1 in, 2 out]
        n6042 = Decrement(x=w13076) -> (x-1=w13080:i32)
        n6043 = Index Array(array=w13077, index=w13080) -> (element=w13078:refnum<vi>)
        n6044 = call "FGV DRV stand.vi"() -> ("Sub-Test.DCV"=w13073:bool)  [unwired: 10 in, 1 out]
        n6045 = call "FGV Driver Data.vi"("DUT index(1-60)"=w13076) -> ("DUT SC"=w13074:bool)  [unwired: 7 in, 3 out]
        n6046 = property class="ColBox"(reference=w13078, "Value"=u32 10000536 ("DRV 1")) -> ()  [unwired: 1 in, 2 out]
        n6047 = case shown="False" w13074 {
          tunnel: w13076 -> [w13094 _]
          tunnel: [w13093 w13159] -> w13075
          tunnel: w13073 -> [w13092 _]
          frame False {
            n6048 = case shown="True" w13092 {
              tunnel: w13094 -> [w13101 w13131]
              tunnel: [w13112 w13130] -> w13093
              frame False {
                w13098 = T9 {"command"="", "data"=variant} ("element")
                w13111 = T9 {"command"="", "data"=variant} ("element")
                n6049 = To Variant(anything=T3."mux10_1_channel6" ("mux10_1(x6)_encode")) -> (Variant=w13109:variant)
                n6050 = To Variant(anything=T4."demux1_10_channel6" ("demux1_10(x6)_encode")) -> (Variant=w13105:variant)
                n6051 = To Variant(anything=bool[] [FALSE, FALSE, TRUE, FALSE, FALSE, FALSE]) -> (Variant=w13120:variant)
                n6052 = Bundle By Name(cluster=w13111, "command"="MEAS.AllRelaysOFF") -> (w13119:T9)
                n6053 = Bundle By Name(cluster=w13111, "command"="MEAS.mux10-1", "data"=w13109) -> (w13102:T9)
                n6054 = Bundle By Name(cluster=w13111, "command"="MEAS.demux1-10", "data"=w13105) -> (w13103:T9)
                n6055 = Bundle By Name(cluster=w13111, "command"="MEAS.eMIC", "data"=w13120) -> (w13104:T9)
                n6056 = Build Array(w13119, w13102, w13103, w13104) -> (w13097:T9[])
                n6057 = To Variant(anything=w13101) -> (Variant=w13100:variant)
                n6058 = To Variant(anything=w13101) -> (Variant=w13099:variant)
                n6059 = Bundle By Name(cluster=w13098, "command"="MEAS.requestAC", "data"=w13100) -> (w13117:T9)
                n6060 = Bundle By Name(cluster=w13098, "command"="Apps.WaitForEvent", "data"=w13099) -> (w13113:T9)
                n6061 = Bundle By Name(cluster=w13098, "command"="Apps.UI Update 1") -> (w13114:T9)
                n6062 = Bundle By Name(cluster=w13098, "command"="WaitFor") -> (w13096:T9)
                n6063 = Build Array (concatenate)(w13097, w13096, w13117, w13113, w13114) -> (w13112:T9[])
              }
              frame True {
                w13127 = T9 {"command"="", "data"=variant} ("element")
                w13149 = T9 {"command"="", "data"=variant} ("element")
                n6064 = To Variant(anything=T3."mux10_1_channel6" ("mux10_1(x6)_encode")) -> (Variant=w13156:variant)
                n6065 = To Variant(anything=T2."mux6_1_channel3_3" ("mux6_1(3wires)_encode")) -> (Variant=w13154:variant)
                n6066 = To Variant(anything=T4."demux1_10_channel6" ("demux1_10(x6)_encode")) -> (Variant=w13150:variant)
                n6067 = To Variant(anything=bool[] [FALSE, FALSE, TRUE, FALSE, FALSE, FALSE]) -> (Variant=w13146:variant)
                n6068 = Bundle By Name(cluster=w13149, "command"="MEAS.AllRelaysOFF") -> (w13145:T9)
                n6069 = Bundle By Name(cluster=w13149, "command"="MEAS.mux10-1", "data"=w13156) -> (w13144:T9)
                n6070 = Bundle By Name(cluster=w13149, "command"="MEAS.mux6_1", "data"=w13154) -> (w13143:T9)
                n6071 = Bundle By Name(cluster=w13149, "command"="MEAS.demux1-10", "data"=w13150) -> (w13142:T9)
                n6072 = Bundle By Name(cluster=w13149, "command"="MEAS.eMIC", "data"=w13146) -> (w13141:T9)
                n6073 = Build Array(w13145, w13144, w13143, w13142, w13141) -> (w13126:T9[])
                n6074 = To Variant(anything=w13131) -> (Variant=w13129:variant)
                n6075 = To Variant(anything=w13131) -> (Variant=w13128:variant)
                n6076 = Bundle By Name(cluster=w13127, "command"="WaitFor") -> (w13125:T9)
                n6077 = Bundle By Name(cluster=w13127, "command"="MEAS.DMM dual read") -> (w13138:T9)
                n6078 = Bundle By Name(cluster=w13127, "command"="MEAS.requestAC", "data"=w13129) -> (w13137:T9)
                n6079 = Bundle By Name(cluster=w13127, "command"="Apps.WaitForEvent", "data"=w13128) -> (w13132:T9)
                n6080 = Bundle By Name(cluster=w13127, "command"="Apps.UI Update 1") -> (w13133:T9)
                n6081 = Build Array (concatenate)(w13126, w13125, w13138, w13137, w13132, w13133) -> (w13130:T9[])
              }
            }
          }
          frame True {
            n6082 = Bundle By Name(cluster=T9 {"command"="", "data"=variant} ("element"), "command"="Apps.UI Update 1") -> (w13160:T9)
            n6083 = Build Array(w13160) -> (w13159:T9[])
          }
        }
        n6084 = for {
          tunnel: w13075 -> [w13170] mode=indexing
          tunnel: w13083 -> [w13171]
          tunnel: [w13167] -> w13085 mode=indexing
          n6085 = Unbundle By Name(w13170) -> ("command"=w13169:string, "data"=w13168:variant)
          n6086 = call "App enquece.vi"("command data"=w13168, "command"=w13169, "queue in"=w13171) -> ("error out"=w13167:errorcluster)  [unwired: 7 in, 1 out]
        }
        n6087 = Merge Errors(w13086, w13085) -> (w13084:errorcluster)
      }
      frame "Test DRV 34A" {
        w13175 = 34 ("DUT index(0-59)")
        n6088 = disable-structure shown="LOGGING==TRUE" {
          disable-tunnel: w13180 -> [w13263 _]
          frame condition #0 (active) {
            n6089 = Empty String/Path?(string/path=w13263) -> (empty?=w13265:bool)
            n6090 = Select(t="Quece timeout", s=w13265, f=w13263) -> (s? t:f=w13262:string)
            n6091 = call "string log (SubVI).vi"("state Name"=w13262) -> ()  [unwired: 9 in, 2 out]
          }
          frame condition #1 {
          }
        }
        n6092 = Flush Queue(queue=w13181) -> (queue out=w13182:refnum<queue>)  [unwired: 1 in, 2 out]
        n6093 = Decrement(x=w13175) -> (x-1=w13179:i32)
        n6094 = Index Array(array=w13176, index=w13179) -> (element=w13177:refnum<vi>)
        n6095 = call "FGV DRV stand.vi"() -> ("Sub-Test.DCV"=w13172:bool)  [unwired: 10 in, 1 out]
        n6096 = call "FGV Driver Data.vi"("DUT index(1-60)"=w13175) -> ("DUT SC"=w13173:bool)  [unwired: 7 in, 3 out]
        n6097 = property class="ColBox"(reference=w13177, "Value"=u32 10000536 ("DRV 1")) -> ()  [unwired: 1 in, 2 out]
        n6098 = case shown="False" w13173 {
          tunnel: w13175 -> [w13193 _]
          tunnel: [w13192 w13258] -> w13174
          tunnel: w13172 -> [w13191 _]
          frame False {
            n6099 = case shown="False" w13191 {
              tunnel: w13193 -> [w13200 w13230]
              tunnel: [w13211 w13229] -> w13192
              frame False {
                w13197 = T9 {"command"="", "data"=variant} ("element")
                w13210 = T9 {"command"="", "data"=variant} ("element")
